vi "Test shm get Event applied Settings Match Start LV.vi"(8 "error in (no error)":errorcluster, 11 "logevent_appliedSettingsMatchStart_Ctl":T1) -> (0 "error out":errorcluster, 2 "function return":i32, 3 "logevent_appliedSettingsMatchStart_Ctl out":T1)   [LabVIEW 2018, in "SALLV_Test.lvlib"]
doc: "int Test_shm_getEvent_appliedSettingsMatchStartLV(Test_logevent_appliedSettingsMatchStartLV *logevent_appliedSettingsMatchStart_Ctl );"
uses:
  SALLV_Test.lvlib
  SALLV_Test.so
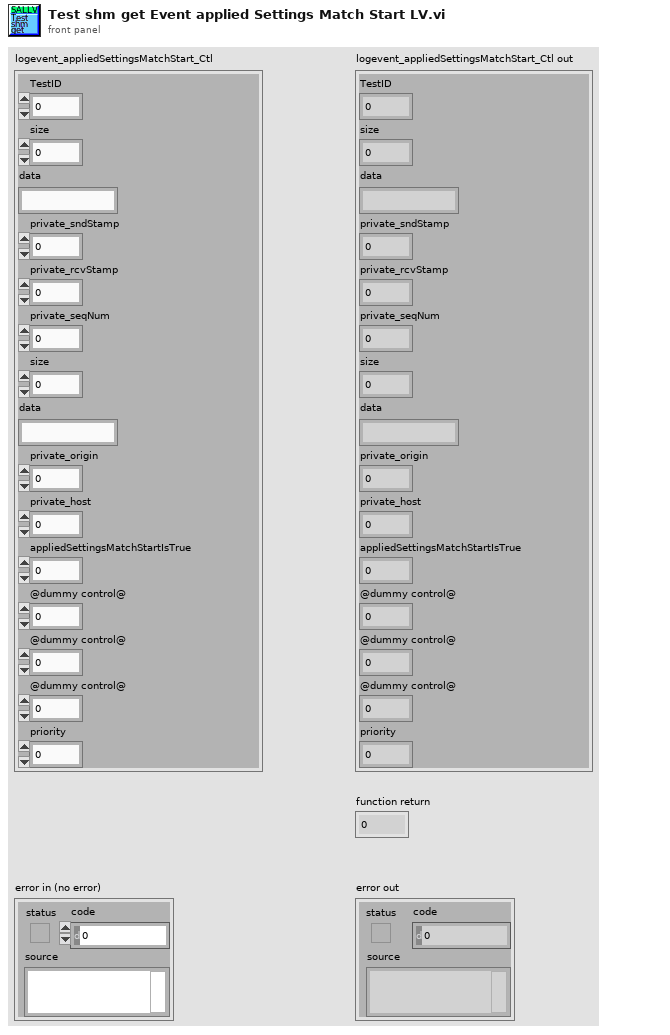
[diagram p1: front panel]
types:
  T1 = cluster{"TestID":i32, "size":i32, "data":string, "private_sndStamp":dbl, "private_rcvStamp":dbl, "private_seqNum":i32, "size":i32, "data":string, "private_origin":i32, "private_host":i32, "appliedSettingsMatchStartIsTrue":u8, "@dummy control@":i8, "@dummy control@":i8, "@dummy control@":i8, "priority":i32}
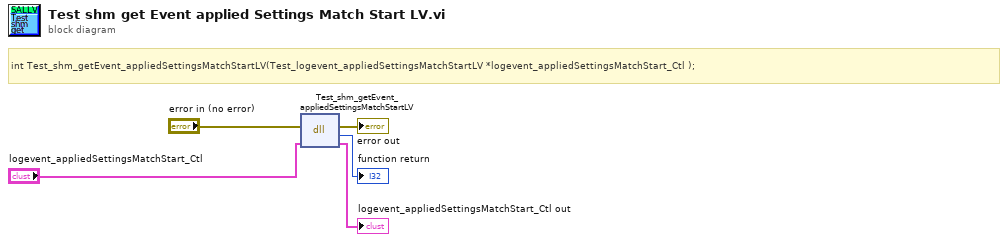
[diagram p0: block diagram]
diagram:
  # "int Test_shm_getEvent_appliedSettingsMatchStartLV(Test_logevent_appliedSettingsMatchStartLV *logevent_appliedSettingsMatchStart_Ctl );"
  n1 = dll-call lib="home/ttsai/Documents/salTestLabViewApi/SALLV_Test/SALLV_Test.*" fn="Test_shm_getEvent_appliedSettingsMatchStartLV"(error in="error in (no error)", "logevent_appliedSettingsMatchStart_Ctl"="logevent_appliedSettingsMatchStart_Ctl") -> (error out=→"error out":errorcluster, →"function return":i32, "logevent_appliedSettingsMatchStart_Ctl"=→"logevent_appliedSettingsMatchStart_Ctl out":T1)  [unwired: 2 in, 1 out]
